vi "Get VI Images.vi"(8 "Error In":errorcluster, 10 "VI Path":path, 11 "Doc Config":T1) -> (0 "Error Out":errorcluster, 1 "BD_Img_Path":string, 2 "Con_Img_Path":string, 3 "Doc Config":T1)   [LabVIEW 2011, in "LMH-Toolbox.lvlib" / "LMH-Documentation.lvlib"]
uses:
  LMH-Documentation.lvlib
  Type Defs/Doc Config.ctl
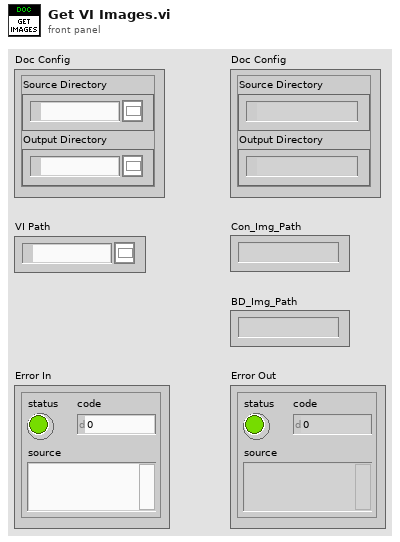
[diagram p1: front panel]
types:
  T1 = typedef "LMH-Toolbox.lvlib/LMH-Documentation.lvlib/Doc Config.ctl" = cluster{"Source Directory":path, "Output Directory":path}
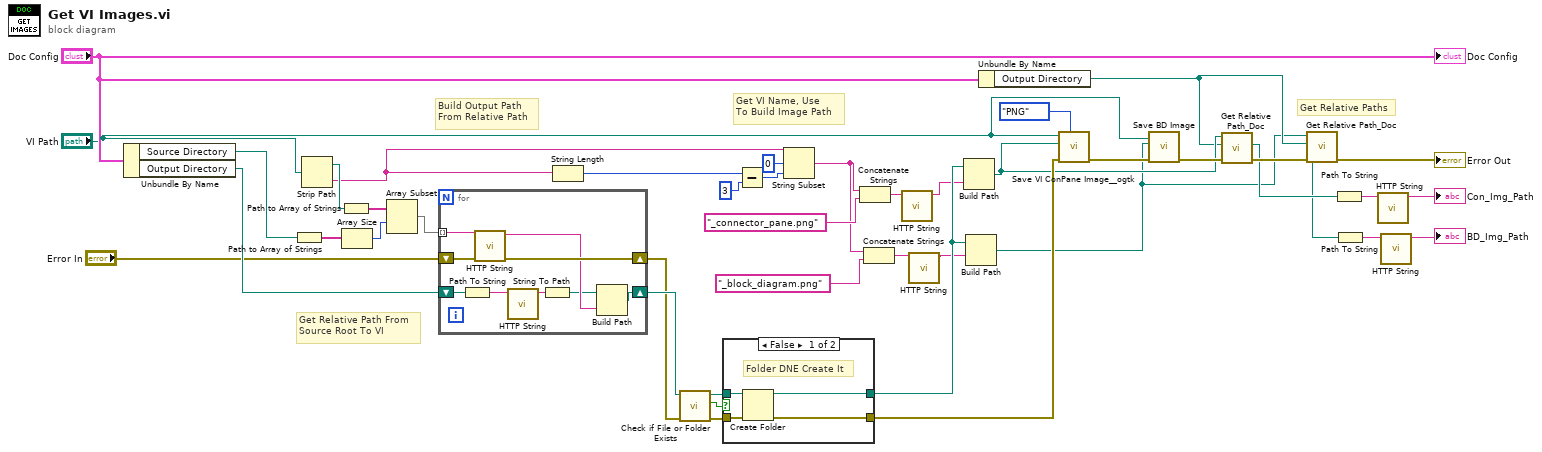
[diagram p0: block diagram]
diagram:
  # "Get Relative Paths"
  # "Get VI Name, Use \nTo Build Image Path"
  # "Build Output Path\nFrom Relative Path"
  # "Get Relative Path From\nSource Root To VI"
  n1 = Unbundle By Name("Doc Config") -> ("Source Directory"=w43:path, "Output Directory"=w42:path)
  n2 = Path to Array of Strings(0:w43) -> (2:w38:string[])  [unwired: 1 out]
  n3 = Strip Path(path="VI Path") -> (stripped path=w36:path, name=w35:string)
  n4 = Path to Array of Strings(0:w36) -> (2:w39:string[])  [unwired: 1 out]
  n5 = Array Size(array=w38) -> (size(s)=w40:i32)
  n6 = Array Subset(array=w39, index=w40) -> (w37:string[])  [unwired: 1 in]
  n7 = for {
    tunnel: w37 -> [w49] mode=indexing
    shift-right: [w52] -> w26
    shift-left: w42 -> [w46]
    shift-right: [w50] -> w6
    shift-left: "Error In" -> [w51]
    n8 = Path To String(path=w46) -> (string=w47:string)
    n9 = call "HTTP String.vi"("Error In"=w51, "String in"=w49) -> ("Error Out"=w50:errorcluster, "String out"=w48:string)  [unwired: 8 in]
    n10 = call "HTTP String.vi"("String in"=w47) -> ("String out"=w45:string)  [unwired: 9 in, 1 out]
    n11 = String To Path(string=w45) -> (path=w44:path)
    n12 = Build Path(base path=w44, name or relative path=w48) -> (appended path=w52:path)
  }
  n13 = String Length(string=w35) -> (length=w34:i32)
  n14 = call <vilib>:"Check if File or Folder Exists.vi"("error in (no error)"=w6, "path"=w26) -> ("error out"=w28:errorcluster, "file or folder exists?"=w29:bool, "dup path"=w30:path)  [unwired: 7 in]
  n15 = case shown="False" w29 {
    tunnel: [w54 w58] -> w27
    tunnel: w28 -> [w56 w58]
    tunnel: w30 -> [w55 w57]
    tunnel: [w53 w57] -> w19
    frame False {
      # "Folder DNE Create It"
      n16 = Create Folder(path (use dialog)=w55, error in=w56) -> (created path=w53:path, error out=w54:errorcluster)  [unwired: 1 in, 1 out]
    }
    frame True {
    }
  }
  n17 = Subtract(x=w34, y=3) -> (x-y=w32:i32)
  n18 = String Subset(string=w35, offset (0)=0, length (rest)=w32) -> (substring=w20:string)
  n19 = Concatenate Strings(w20, "_connector_pane.png" ("string")) -> (w4:string)
  n20 = Concatenate Strings(w20, "_block_diagram.png" ("string")) -> (w2:string)
  n21 = call "HTTP String.vi"("String in"=w4) -> ("String out"=w3:string)  [unwired: 9 in, 1 out]
  n22 = call "HTTP String.vi"("String in"=w2) -> ("String out"=w1:string)  [unwired: 9 in, 1 out]
  n23 = Build Path(base path=w19, name or relative path=w3) -> (appended path=w17:path)
  n24 = Build Path(base path=w19, name or relative path=w1) -> (appended path=w12:path)
  n25 = Unbundle By Name("Doc Config") -> ("Output Directory"=w15:path)
  n26 = call <userlib>:"Save VI ConPane Image__ogtk.vi"("Image Format"=enum32{"PNG", "JPEG", "GIF"}."PNG", "error in (no error)"=w27, "Image File Path"=w17, "VI Path"="VI Path") -> ("error out"=w24:errorcluster)  [unwired: 7 in]
  n27 = call "Save BD Image.vi"("Error In"=w24, "Target BD Image Path"=w12, "VI Path"="VI Path") -> ("Error Out"=w18:errorcluster)  [unwired: 8 in]
  n28 = call "Get Relative Path_Doc.vi"("Error In"=w18, "Relative Path Root"=w15, "File / Folder"=w17) -> ("Error Out"=w16:errorcluster, "Relative Path"=w14:path)  [unwired: 6 in, 1 out]
  n29 = call "Get Relative Path_Doc.vi"("Error In"=w16, "Relative Path Root"=w15, "File / Folder"=w12) -> ("Error Out"=→"Error Out":errorcluster, "Relative Path"=w13:path)  [unwired: 6 in, 1 out]
  n30 = Path To String(path=w14) -> (string=w10:string)
  n31 = Path To String(path=w13) -> (string=w8:string)
  n32 = call "HTTP String.vi"("String in"=w10) -> ("String out"=→"Con_Img_Path":string)  [unwired: 9 in, 1 out]
  n33 = call "HTTP String.vi"("String in"=w8) -> ("String out"=→"BD_Img_Path":string)  [unwired: 9 in, 1 out]
  "Doc Config" <- "Doc Config"
